vi "Search Timer By Name.vi"(8 "error in (no error)":errorcluster, 10 "Name":string, 11 "Array":refnum<class "Timer.lvclass">[](array[class])) -> (0 "error out":errorcluster, 1 "index of element":i32, 2 "element":refnum<class "Timer.lvclass">, 3 "Array 2":refnum<class "Timer.lvclass">[](array[class]))   [LabVIEW 2017, in "TimerEngine.lvlib" / "Timer.lvclass"]
uses:
  Timer.lvclass
  Timer.lvclass/Timer.ctl
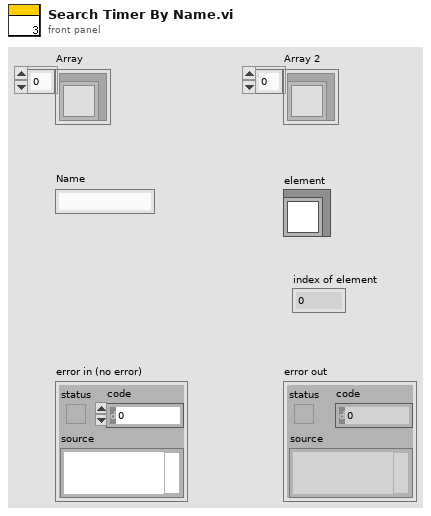
[diagram p1: front panel]
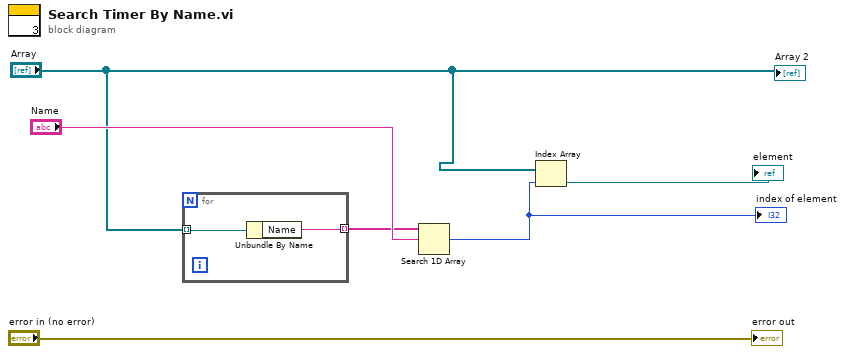
[diagram p0: block diagram]
diagram:
  n1 = for {
    tunnel: "Array" -> [w8] mode=indexing
    tunnel: [w7] -> w4 mode=indexing
    n2 = Unbundle By Name(w8) -> ("Name"=w7:string)
  }
  n3 = Search 1D Array(1D array=w4, element="Name") -> (index of element=w1:i32)  [unwired: 1 in]
  "index of element" <- w1
  n4 = Index Array(array="Array", index=w1) -> (element=→"element":refnum<class "Timer.lvclass">)
  "error out" <- "error in (no error)"
  "Array 2" <- "Array"
